vi "Generator&oscilloscope_final2.vi"() -> ()   [LabVIEW 2018]
uses:
  <instrlib>/LeCroy Wave Series/Public/Data/Read Single Waveform.vi
  <instrlib>/Siglent SDG X Series/Siglent SDG X Series.lvlib
  <instrlib>/LeCroy Wave Series/LeCroy Wave Series.lvlib
panel:
  in  "Tab Control":enum32{"Page 1", "Page 2"}(tab)
  in  "VISA Refnum in":refnum<visa-resource-name>="USB0::0xF4EC::0xEE38::SDG2XCAD2R3765::INSTR"
  in  "Channel (1:Channel 1)":i32(ring)=1 items=["Channel 1"=1, "Channel 2"=2]
  in  "Enable Output (T: Enable)":bool=TRUE
  in  "Amplitude (1.0 Vpp)":dbl=1.0 format="%#.3f"
  in  "Frequency (1000 Hz)":dbl=1000.0 format="%#.6g"
  in  "DC Offset (0.00 V) in":dbl
  in  "Waveform Function (0: Sine) in":u16(ring) items=["Sine", "Square", "Ramp", "DC", "Pulse", "Arb"]
  in  "Phase (0.0 degrees)":dbl=0.002 min=-360.0 max=360.0 format="%#.1g"
  in  "Fall (20 ns)":dbl=2e-08 format="%#.3g"
  in  "Duty (20%)":dbl=20.0 min=0.0001 max=100.0 format="%.4g"
  in  "Delay (0.00 s)":dbl min=-1000000.0 max=1000000.0
  in  "Rise (20 ns)":dbl=2e-08 format="%#.3g"
  in  "True To \ngenerate\n pulse":bool
  out "VISA resource name out":refnum<visa-resource-name>
  out "error out":errorcluster
  in  "format string":string="Channel: %g \nWavetype: %g \nAMP: %gV\nFreq: %gHz \nRiseTime: %gs \nFallTime: %gs \nDutyCycle: %g"
  out "Output Filename":path
  out "error out 2":errorcluster
  out "Output Directory":path
  in  "File Directory":path
  in  "Filename":string
  out ".not. x?":bool
  in  "stop":bool
  out "Waveform Data":waveform(dbl)(graph)
  in  "Timeout (10000 ms)":u32=10000
  in  "Source (0: Channel 1)":u16(ring) items=["Channel 1", "Channel 2", "Channel 3", "Channel 4", "Memory 1", "Memory 2", "Memory 3", "Memory 4", "Function 1", "Function 2", "Function 3", "Function 4", "Function 5", "Function 6", "Function 7", "Function 8"]
  in  "Perform Auto Setup?":bool
  in  "Reset Scope?":bool
  in  "VISA resource name":refnum<visa-resource-name>
  out "Saved filename":string
  in  "Save Files in Directory":string="D:\\Automation\\Data"
  in  "Filename":string="Title"
  in  "Path to save DATA":path=path "E:/Ankur/Labview/Automation/Files/Oscdata"
  # "Set PULSE parameters"
  # "In the oscilloscope memory"
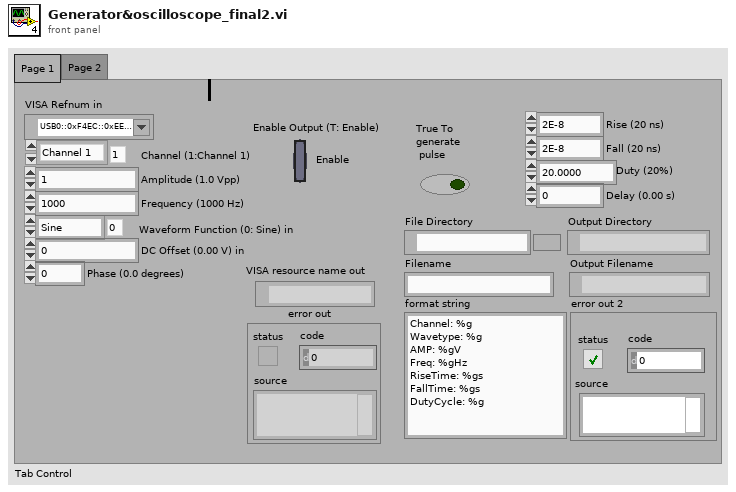
[diagram p1: front panel]
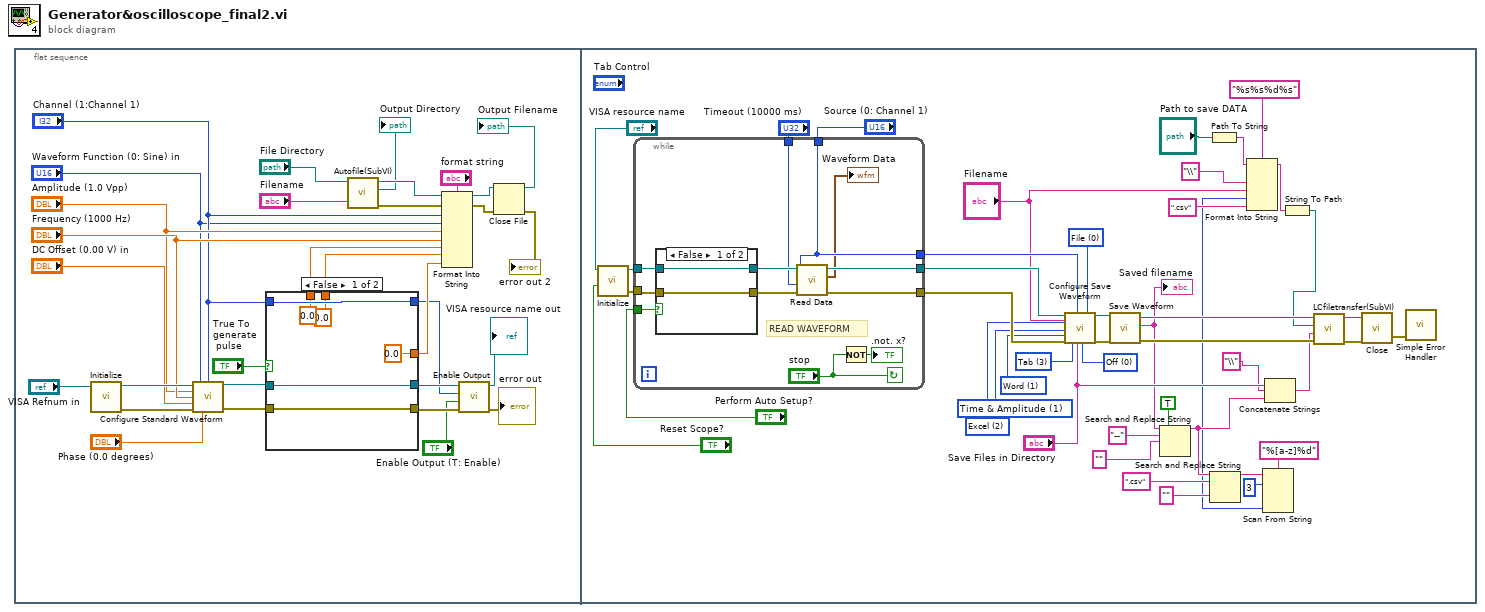
[diagram p0: block diagram]
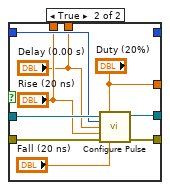
[diagram p2: hidden frame]
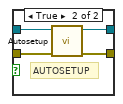
[diagram p3: hidden frame]
diagram:
  n1 = flat-sequence {
    frame #0 {
      n2 = call <instrlib>:"Initialize.vi"("VISA resource name"="VISA Refnum in") -> ("error out"=w25:errorcluster, "VISA resource name out"=w26:refnum<visa-resource-name>)  [unwired: 9 in]
      n3 = call <instrlib>:"Configure Standard Waveform.vi"("VISA resource name"=w26, "Waveform Function (0: Sine)"="Waveform Function (0: Sine) in", "Channel (1:Channel 1)"="Channel (1:Channel 1)", "Amplitude (1.0 Vpp)"="Amplitude (1.0 Vpp)", "Frequency (1000 Hz)"="Frequency (1000 Hz)", "DC Offset (0.00 V)"="DC Offset (0.00 V) in", "error in (no error)"=w25, "Phase (0.0 degrees)"="Phase (0.0 degrees)") -> ("VISA resource name out"=w21:refnum<visa-resource-name>, "error out"=w24:errorcluster)  [unwired: 6 in]
      n4 = case shown="False" "True To \ngenerate\n pulse" {
        tunnel: [w35 w43] -> w30
        tunnel: [w34 w42] -> w29
        tunnel: w21 -> [w35 w41]
        tunnel: w24 -> [w34 w40]
        tunnel: "Channel (1:Channel 1)" -> [_ w39]
        tunnel: "Channel (1:Channel 1)" -> [_ _]
        tunnel: [0.0 ("Duty (20%)") "Duty (20%)"] -> w17
        tunnel: [0.0 ("Rise (20 ns)") "Rise (20 ns)"] -> w9
        tunnel: [0.0 ("Delay (0.00 s)") "Delay (0.00 s)"] -> w8
        frame False {
        }
        frame True {
          n5 = call <instrlib>:"Configure Pulse.vi"("VISA resource name"=w41, "Duty (20%)"="Duty (20%)", "Channel (1:Channel 1)"=w39, "Delay (0.00 s)"="Delay (0.00 s)", "Rise (20 ns)"="Rise (20 ns)", "error in (no error)"=w40, "Fall (20 ns)"="Fall (20 ns)") -> ("VISA resource name out"=w43:refnum<visa-resource-name>, "error out"=w42:errorcluster)  [unwired: 7 in]
        }
      }
      n6 = call "Autofile(SubVI).vi"("Filename"="Filename", "File Directory"="File Directory") -> ("error out"=w4:errorcluster, "Output Directory"=→"Output Directory":path, "Byte Stream File out"=w5:refnum<file>)  [unwired: 7 in]
      n7 = Format Into String(format string="format string", initial string=w5, error in=w4, "Channel (1:Channel 1)", "Waveform Function (0: Sine) in", "Amplitude (1.0 Vpp)", "Frequency (1000 Hz)", w9, w8, w17) -> (resulting string=w16:refnum<file>, error out=w13:errorcluster)
      n8 = call <instrlib>:"Enable Output.vi"("error in (no error)"=w29, "Enable Output (T: Enable)"="Enable Output (T: Enable)", "Channel (1:Channel 1)"="Channel (1:Channel 1)", "VISA resource name"=w30) -> ("error out"=→"error out":errorcluster, "VISA resource name out"=→"VISA resource name out":refnum<visa-resource-name>)  [unwired: 6 in]
      n9 = Close File(refnum=w16, error in=w13) -> (path=→"Output Filename":path, error out=→"error out 2":errorcluster)
    }
    frame #1 {
      w73 = u16 3 items=["Comma", "Space", "Semicolon", "Tab"] ("Delimiter (  0:Comma)")
      w74 = u16 0 items=["Off", "Wrap", "Fill"] ("Auto Save (0:Off")
      w75 = u16 1 items=["Byte", "Word", "Auto"] ("BinarySubFormat (1: Word)")
      w76 = u16 1 items=["Amplitude Only", "Time & Amplitude", "With Header"] ("SubFormat (1: Time & Amplitude)")
      w77 = u16 2 items=["Binary", "ASCII", "Excel", "MATLAB", "MathCad", "WaveML"] ("Format (0: Binary)")
      w78 = u16 0 items=["File", "M1", "M2", "M3", "M4"] ("Destination (0:File)")
      n10 = call <instrlib>:"Initialize.vi"("Reset? (T: Yes)"="Reset Scope?", "VISA resource name"="VISA resource name") -> ("error out"=w86:errorcluster, "VISA resource name out"=w87:refnum<visa-resource-name>)  [unwired: 8 in]
      n11 = while {
        tunnel: [w90] -> w80
        tunnel: [w99] -> w81
        tunnel: "Perform Auto Setup?" -> [w98]
        tunnel: "Source (0: Channel 1)" -> [w92]
        tunnel: w86 -> [w97]
        tunnel: w87 -> [w96]
        tunnel: "Timeout (10000 ms)" -> [w95]
        tunnel: [w92] -> w79
        stop <- "stop" continue-if-true
        # "READ WAVEFORM"
        n12 = case shown="False" w98 {
          tunnel: w97 -> [w102 w107]
          tunnel: w96 -> [w103 w106]
          tunnel: [w103 w105] -> w101
          tunnel: [w102 w104] -> w100
          frame False {
          }
          frame True {
            # "AUTOSETUP"
            n13 = call <instrlib>:"Autosetup.vi"("error in (no error)"=w107, "VISA resource name"=w106) -> ("error out"=w104:errorcluster, "VISA resource name out"=w105:refnum<visa-resource-name>)  [unwired: 8 in]
          }
        }
        n14 = call-poly <instrlib>:"Read Data.vi"("error in (no error)"=w100, "Timeout (10000 ms)"=w95, "Source (0: Channel 1)"=w92, "VISA resource name"=w101) -> ("error out"=w90:errorcluster, "Waveform Data"=→"Waveform Data":waveform(dbl), "VISA resource name out"=w99:refnum<visa-resource-name>)  [unwired: 5 in]
        n15 = Not(x="stop") -> (.not. x?=→".not. x?":bool)
      }
      n16 = call <instrlib>:"Configure Save Waveform.vi"("VISA resource name"=w81, "Trace Title (Title)"="Filename", "Format (0: Binary)"=w77, "SubFormat (1: Time & Amplitude)"=w76, "BinarySubFormat (1: Word)"=w75, "error in (no error)"=w80, "Delimiter (  0:Comma)"=w73, "Source (0: Channel 1)"=w79, "Save Files in Directory (D:\\Waveforms)"="Save Files in Directory", "Auto Save (0:Off"=w74, "Destination (0:File)"=w78) -> ("VISA resource name out"=w72:refnum<visa-resource-name>, "error out"=w71:errorcluster)  [unwired: 7 in]
      n17 = call <instrlib>:"Save Waveform.vi"("error in (no error)"=w71, "VISA resource name"=w72) -> ("error out"=w66:errorcluster, "Saved filename"=w56:string, "VISA resource name out"=w67:refnum<visa-resource-name>)  [unwired: 7 in]
      "Saved filename" <- w56
      n18 = Search and Replace String(replace all?=TRUE ("replace all? (F)"), input string=w56, search string="--", replace string="" ("replace string (\"\")")) -> (result string=w48:string)  [unwired: 4 in, 3 out]
      n19 = Path To String(path="Path to save DATA") -> (string=w54:string)
      n20 = Search and Replace String(input string=w48, search string=".csv", replace string="" ("replace string (\"\")")) -> (result string=w51:string)  [unwired: 5 in, 3 out]
      n21 = Scan From String(format string="%[a-z]%d", input string=w51, initial scan location=u32 3) -> (output 2=w46:i32)  [unwired: 4 in, 3 out]
      n22 = Format Into String(format string="%s%s%d%s", initial string=w54, "\\" ("input 1"), "Filename", w46, ".csv" ("input 3")) -> (resulting string=w60:string)  [unwired: 1 in, 1 out]
      n23 = Concatenate Strings("Save Files in Directory", "\\" ("string"), w48) -> (w65:string)
      n24 = String To Path(string=w60) -> (path=w62:path)
      n25 = call <userlib>:"LCfiletransfer(SubVI).vi"("error in (no error)"=w66, "Source Filename"=w65, "file path (use dialog)"=w62, "VISA Refnum in"=w67) -> ("error out"=w63:errorcluster, "VISA Refnum out"=w64:refnum<visa-resource-name>)  [unwired: 5 in, 1 out]
      n26 = call <instrlib>:"Close.vi"("error in (no error)"=w63, "VISA resource name"=w64) -> ("error out"=w89:errorcluster)  [unwired: 9 in]
      n27 = call <vilib>:"Simple Error Handler.vi"("error in (no error)"=w89) -> ()  [unwired: 4 in, 5 out]
    }
  }
